vi "vew --scan pipe.vi"() -> ()   [LabVIEW 2010]
uses:
  <vilib>/event_ctls.llb/eventvkey.ctl
  cursor window action.ctl
  cursor winow.ctl
  tale of three indices -- int -- control.ctl
  filter method control.ctl
panel:
  in  "filter method":T1
  in  "step once":bool
  out "Numeric":i32
  out "tale of three indices -- int -- control out":T2={"left"=0, "center"=0, "right"=0, "right most"=0, "left most"=0, "window"=0, "max win factor"=2, "max win"=2, "min win"=2}
  out "norm":dbl
  out "center":cdb
  out "Plot: fragment":cluster{dbl[], dbl[]}[](graph)
  in  "smart filter: span":dbl(slide)=0.1 min=0.0001 max=0.5 step=0.001 scale=0.001..0.5 scale format="%#_2g"
  in  "smart filter: delta":dbl(slide)=0.1 min=0.0005 max=0.1 step=0.0001 scale=0.0001..0.1 scale format="%#_2g"
  in  "scale gauge: Plot: complex plane - filter":dbl(slide)=0.3 min=0.0 max=0.3 step=1e-05 scale=1e-05..0.3 scale format="%#_2g"
  out "Plot: complex plane - filter":cluster{dbl[], dbl[]}[](graph)=[{array[1630 elements], array[1630 elements]}, {[0.4066553079816637, 0.40327728987953354, 0.3931965089365436, 0.37657194509013175, 0.35366577764318885, 0.3248392505398343, 0.2905469753326207, 0.2513297616867779, 0.20780608848872892, 0.16066235006458904, 0.11064203133161113, 0.058533982596904274, 0.005159978916854432, -0.048638239786419776, -0.10201224346646971, -0.15412029220117648, -0.20414061093415437, -0.25128434935829436, -0.29480802255634325, -0.33402523620218605, -0.36831751140939956, -0.39714403851275415, -0.4200502059596971, -0.4366747698061089, -0.44675555074909884, -0.450133568851229, -0.44675555074909884, -0.4366747698061089, -0.420050205959697, -0.3971440385127541, -0.3683175114093995, -0.334025236202186, -0.29480802255634314, -0.25128434935829413, -0.20414061093415412, -0.15412029220117648, -0.10201224346646963, -0.04863823978641969, 0.005159978916854609, 0.05853398259690454, 0.11064203133161105, 0.160662350064589, 0.207806088488729, 0.25132976168677806, 0.2905469753326208, 0.3248392505398345, 0.35366577764318885, 0.3765719450901318, 0.3931965089365437, 0.40327728987953354], [-0.02173913043478265, 0.03195292977291478, 0.08479823411705473, 0.1359633805798755, 0.18464146423708142, 0.23006480263052065, 0.27151704257914155, 0.30834445749658657, 0.33996625704997624, 0.36588374657040623, 0.3856881917657815, 0.399067264704769, 0.40580996941485, 0.40580996941485, 0.39906726470476894, 0.3856881917657815, 0.36588374657040623, 0.33996625704997624, 0.30834445749658657, 0.2715170425791415, 0.23006480263052065, 0.18464146423708136, 0.1359633805798754, 0.08479823411705474, 0.03195292977291471, -0.02173913043478279, -0.07543119064248009, -0.12827649498662014, -0.17944164144944094, -0.22811972510664674, -0.273543063500086, -0.31499530344870685, -0.3518227183661519, -0.38344451791954165, -0.40936200743997164, -0.4291664526353468, -0.4425455255743343, -0.4492882302844153, -0.4492882302844153, -0.44254552557433424, -0.42916645263534686, -0.40936200743997153, -0.38344451791954154, -0.3518227183661518, -0.3149953034487067, -0.27354306350008567, -0.22811972510664671, -0.17944164144944075, -0.12827649498661992, -0.07543119064247988]}, {[-0.08588521013843603, -0.0794706021680707, -0.07305599419770535, -0.06664138622734002, -0.06022677825697468, -0.05381217028660934, -0.04739756231624401, -0.04098295434587867, -0.03456834637551333, -0.02815373840514799, -0.02173913043478265, -0.015324522464417317, -0.008909914494051985, -0.0024953065236866384, 0.003919301446678694, 0.01033390941704404, 0.016748517387409373, 0.023163125357774705, 0.029577733328140052, 0.035992341298505384], [0.4018255934561417, 0.35946912106704926, 0.31711264867795685, 0.2747561762888644, 0.23239970389977196, 0.19004323151067953, 0.14768675912158707, 0.10533028673249467, 0.06297381434340221, 0.020617341954309754, -0.02173913043478265, -0.06409560282387511, -0.10645207521296757, -0.14880854760206003, -0.19116501999115237, -0.23352149238024483, -0.2758779647693373, -0.31823443715842975, -0.3605909095475222, -0.40294738193661456]}, {[0.4018255934561417, 0.35946912106704926, 0.31711264867795685, 0.2747561762888644, 0.23239970389977196, 0.19004323151067953, 0.14768675912158707, 0.10533028673249467, 0.06297381434340221, 0.020617341954309754, -0.02173913043478265, -0.06409560282387511, -0.10645207521296757, -0.14880854760206003, -0.19116501999115237, -0.23352149238024483, -0.2758779647693373, -0.31823443715842975, -0.3605909095475222, -0.40294738193661456], [0.04240694926887073, 0.03599234129850539, 0.029577733328140055, 0.02316312535777472, 0.01674851738740938, 0.01033390941704404, 0.003919301446678708, -0.0024953065236866315, -0.008909914494051971, -0.01532452246441731, -0.02173913043478265, -0.028153738405147982, -0.034568346375513315, -0.04098295434587866, -0.047397562316243994, -0.05381217028660934, -0.06022677825697467, -0.06664138622734, -0.07305599419770535, -0.07947060216807068]}, {[-0.03480491194516355, -0.03153571549706419, -0.02826039650219348, -0.024981001928307045, -0.021699581290264596, -0.018418185369150124, -0.015138864930600241, -0.011863669443142526, -0.008594645797344487, -0.0053338370265733695, -0.002083281030167059, 0.0011549907001868857, 0.004378954350067313, 0.007586595047137542, 0.010775908120375176, 0.01394490035292599, 0.017091591227799845, 0.020214014165629166, 0.023310217753717, 0.02637826696560664], [-0.15235728022815603, -0.15264307469559787, -0.15284705845898403, -0.15296910403510236, -0.15300913514944053, -0.15296712678385516, -0.15284310519220728, -0.1526371478839546, -0.15234938357571062, -0.15197999211080082, -0.15152920434686656, -0.15099730201158656, -0.15038461752660615, -0.14969153379978473, -0.1489184839858907, -0.1480659512158939, -0.1471344682950244, -0.1461246173697867, -0.14503702956413708, -0.14387238458505142]}, {[-0.03913246135316176, -0.03478046636428151, -0.030420320964959106, -0.026054750104140326, -0.021686482121507648, -0.017318247042357023, -0.012952774871420701, -0.008592793886703221, -0.004241028934396603, 9.980027406010505e-05, 0.00442698086171163, 0.008737808481546538, 0.013029589006625965, 0.017299640213825143, 0.021545293460135825, 0.02576389535048096, 0.02995280939600055, 0.03410941766177122, 0.038231122402930216, 0.04231534768818167], [-0.19561963666378376, -0.19600008981485692, -0.19627163553875665, -0.19643410412824466, -0.19648739404574114, -0.19643147198678232, -0.19626637290083468, -0.19599219996945272, -0.19560912454179388, -0.1951173860275308, -0.19451729174722807, -0.19380921674027698, -0.19299360353050807, -0.1920709618496281, -0.1910418683186543, -0.1899069660875451, -0.18866696443325223, -0.1873226383164459, -0.18587482789718943, -0.1843244380098665]}]
  in  "create bin file from dat":bool=TRUE
  in  "# columns in bin file":i32=3
  in  "read freq in":bool=TRUE
  in  "filter window (kHz)":dbl=40.0 caption="(kHz)"
  out "all:max omega":dbl=3099.911666666456
  out "all:min omega":dbl=450.0
  in  "filter  all":bool
  in  "phase is normalized":bool=TRUE
  out "Plot: All":cluster{"all rows":dbl[], "all rows":dbl[]}[](graph)
  in  "cursor bracket: All, data window":T3={"left"=2889.388009121066, "right "=2961.3698154668923, "center"=2923.047912677266, "window"=71.98180634582651, "cursors"=[0, 1, 2], "relative"=1, "absolute"=1, "fixed vertical offset"=2421.6740576496672, "vertical offset"=2421.6740576496672, "skew"=0.0, "default window frac"=0.0, "kind"=enum."symmetric", "skew.left"=0.3, "skew.right"=1.0, "Plot ref"=refnum, "wing order"=enum."back"}
  out "filter w (kHz)":dbl
  out "Char":i16
  in  "file path":path=path "C:/data/RUS/Experiment/ProbeTest/Probe10/Hg1201-4-C199-80K-1/Sweep1/March_2012/032212/201.57400K_900_2100_001_032212.bin"
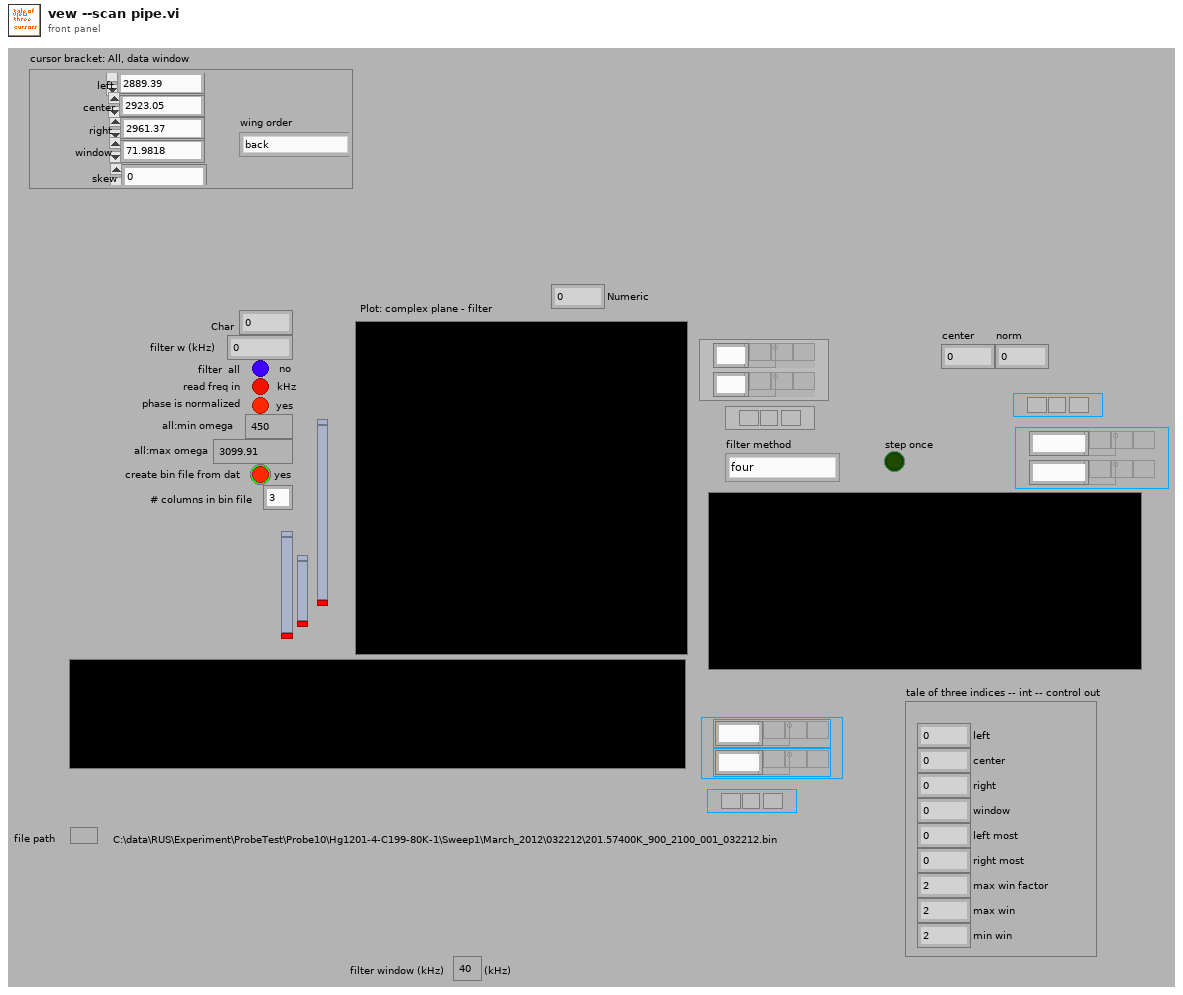
[diagram p1: front panel]
types:
  T1 = typedef "filter method control.ctl" = enum16{"four", "five", "one", "two", "three", "zero", "minus one", "minus two"}
  T2 = typedef "tale of three indices -- int -- control.ctl" = cluster{"left":i32, "center":i32, "right":i32, "right most":i32, "left most":i32, "window":i32, "max win factor":i32, "max win":i32, "min win":i32}
  T3 = typedef "cursor winow.ctl" = cluster{"left":dbl, "right ":dbl, "center":dbl, "window":dbl, "cursors":i32[], "relative":i32, "absolute":i32, "fixed vertical offset":dbl, "vertical offset":dbl, "skew":dbl, "default window frac":dbl, "kind":enum16{"symmetric", "skewed", "fancy"}, "skew.left":dbl, "skew.right":dbl, "Plot ref":refnum<vi>, "wing order":enum16{"forw", "back"}}
  T4 = typedef "eventvkey.ctl" = enum16{"ASCII", "Enter", "Return", "Shift", "Ctrl", "Alt", "Cmd", "Opt", "Caps", "NumLock", "Clear", "Break", "Up", "Down", "Left", "Right", "Insert", "Delete", "Home", "End", "PageUp", "PageDown", "Escape", "Help", "Pause", "ScrollLock", "F1", "F2", "F3", "F4", "F5", "F6", "F7", "F8", "F9", "F10", "F11", "F12", "F13", "F14", "F15", "F16", "F17", "F18", "F19", "F20", "F21", "F22", "F23", "F24", "Play", "VolumeUp", "VolumeDown", "Mute", "Two Byte Char"}
  T5 = typedef "cursor window action.ctl" = enum16{"balance", "h. offset change", "cursor moves", "change center", "change window", "init", "check", "reset", "set y to middle", "idle", "-write all Y", "-write left.X", "-write center.X", "-write right.X", "-write all X", "-change center", "-change window", "-change skew", "-read cursor 2", "-read cursor 1", "-read cursor 0", "-read all cursors", "-reset", "-read plot scale", "-set y to middle", "-Q: center.Y is visible", "-Q: window is visible", "-parse center.Y", "-right left from center", "-left move", "-right move", "-set center.Y", "-empty", "-set cursors to default", "-check", "-write center.Y", "-copy cursor 1", "-copy cursor 0", "-copy cursor 2", "move right", "move left", "shrink", "broaden", "skew up", "skew down", "-write plot scale", "zoom X", "change cen&win"}
  T6 = cluster{"left":dbl, "right ":dbl, "center":dbl, "window":dbl, "cursors":i32[], "relative":i32, "absolute":i32, "fixed vertical offset":dbl, "vertical offset":dbl, "skew":dbl, "default window frac":dbl, "kind":enum16{"symmetric", "skewed", "fancy"}, "skew.left":dbl, "skew.right":dbl, "Plot ref":refnum<vi>, "wing order":enum16{"forw", "back"}}
  T7 = typedef "lveventtype.ctl" = enum32{"Null", "Timeout", "App Instance Close", "App Instance Close?", "Autoscale Range Change", "Cell Edit", "Cell Edit?", "Cursor Grab", "Cursor Grab?", "Cursor Move", "Cursor Release", "Data Change", "Direction Change", "Display State Change", "Drag Ended", "Drag Enter", "Drag Leave", "Drag Over", "Drag Source Update", "Drag Starting", "Drag Starting?", "Drop", "Exec State Change", "Key Down", "Key Down?", "Key Repeat", "Key Repeat?", "Key Up", "Listbox Double Click", "Menu Activation?", "Menu Selection (App)", "Menu Selection? (App)", "Menu Selection (User)", "Mouse Down", "Mouse Down?", "Mouse Enter", "Mouse Leave", "Mouse Move", "Mouse Up", "NI Security User Change (App)", "Pane Size", "Panel Close", "Panel Close?", "Panel Resize", "Plot Attribute Change", "Scale Range Change", "Shortcut Menu Activation?", "Shortcut Menu Selection (App)", "Shortcut Menu Selection? (App)", "Shortcut Menu Selection (User)", "Tree Double Click", "Tree Drag", "Tree Drag?", "Tree Drop", "Tree Drop?", "Tree Item Close", "Tree Item Close?", "Tree Item Open", "Tree Item Open?", "Value Change"}
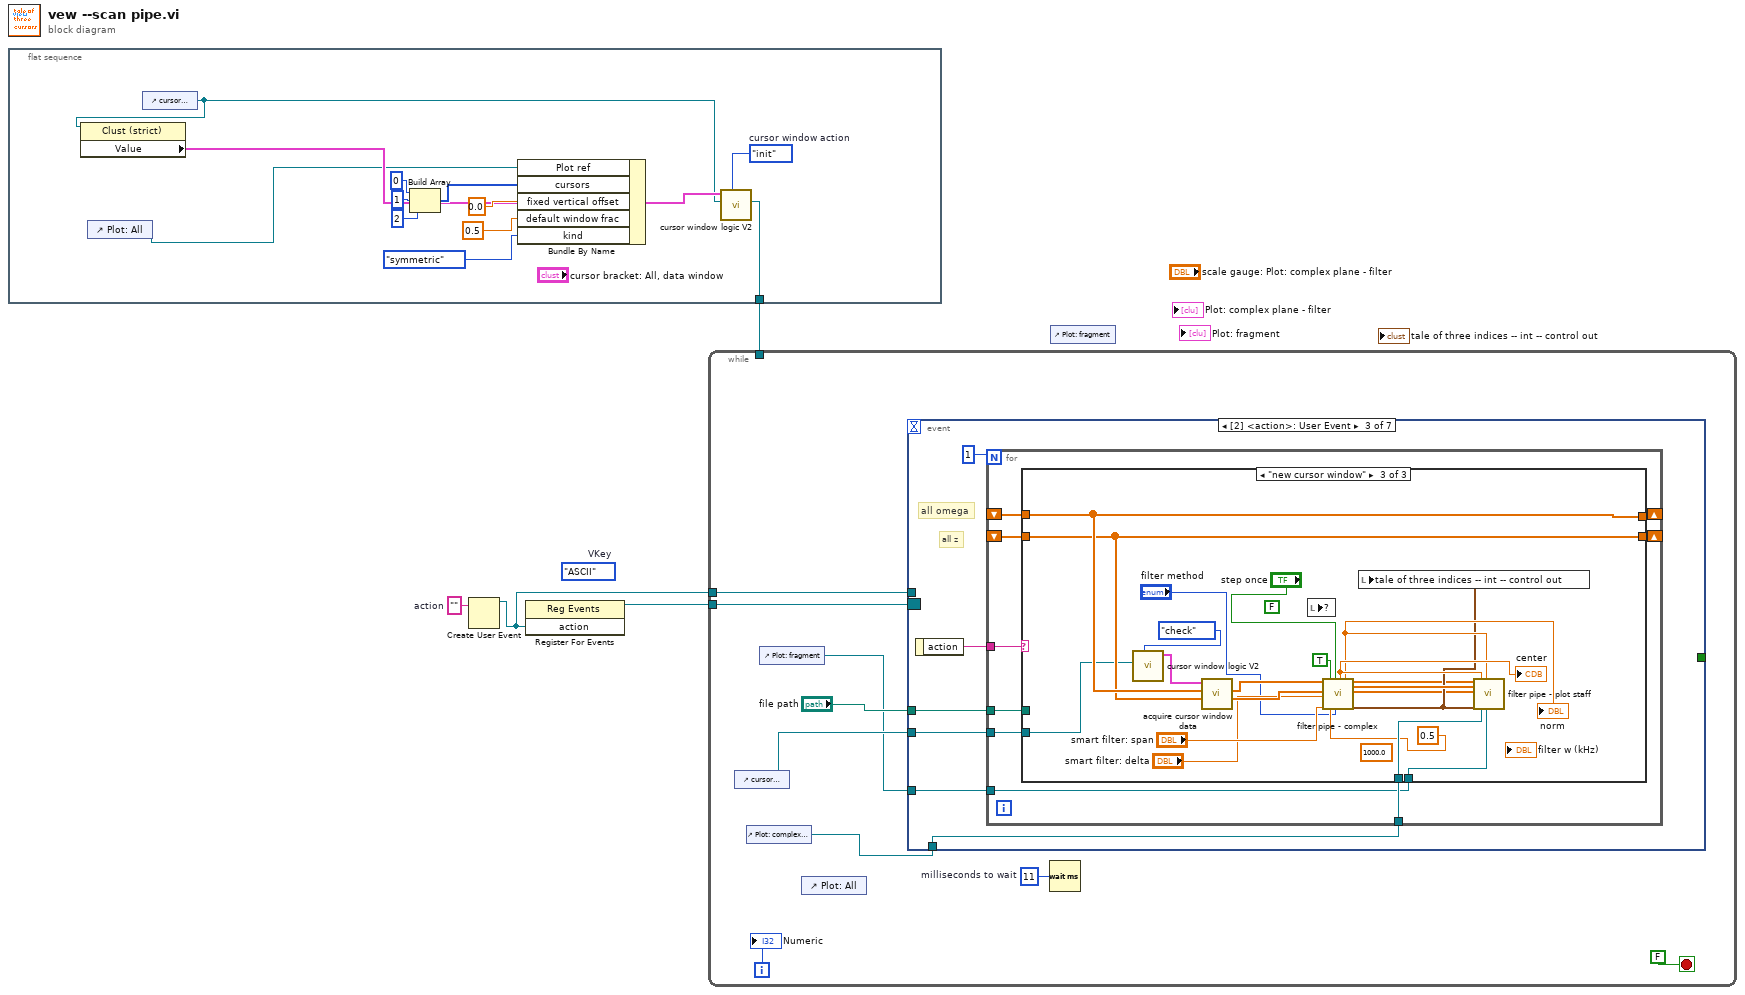
[diagram p0: block diagram]
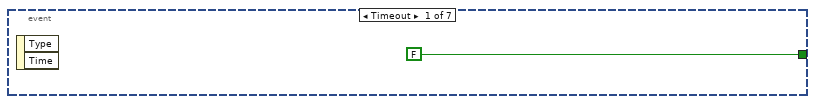
[diagram p2: hidden frame]
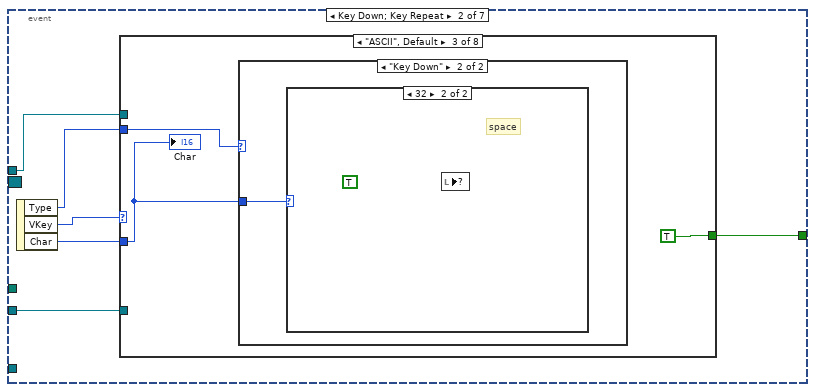
[diagram p3: hidden frame]
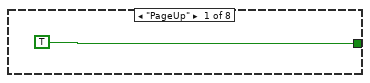
[diagram p4: hidden frame]
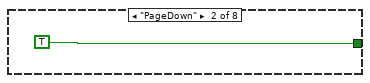
[diagram p5: hidden frame]
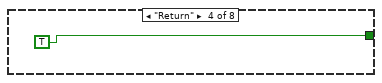
[diagram p8: hidden frame]
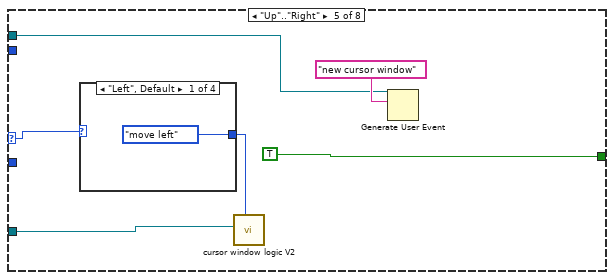
[diagram p9: hidden frame]
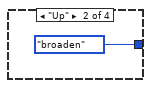
[diagram p10: hidden frame]
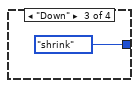
[diagram p11: hidden frame]
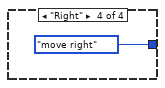
[diagram p12: hidden frame]
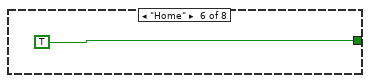
[diagram p13: hidden frame]
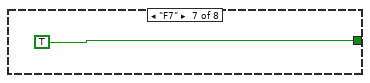
[diagram p14: hidden frame]
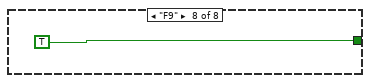
[diagram p15: hidden frame]
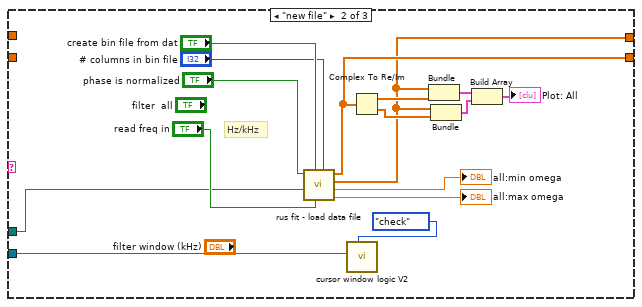
[diagram p17: hidden frame]
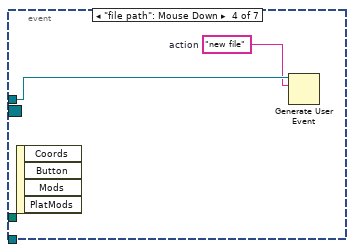
[diagram p18: hidden frame]
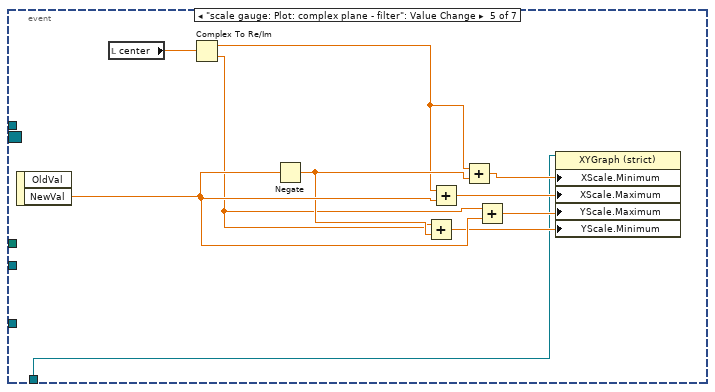
[diagram p19: hidden frame]
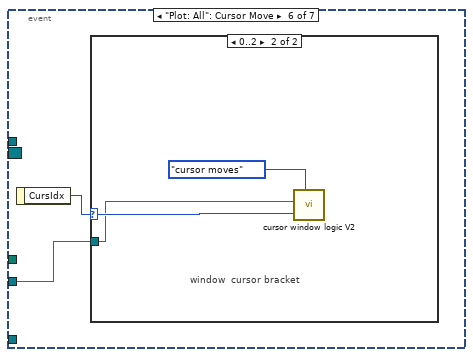
[diagram p20: hidden frame]
diagram:
  (unwired) eventvkey."ASCII"  # VKey
  w3 = ""  # action
  n1 = flat-sequence {
    tunnel: [w5] -> w2
    frame #0 {
      w8 = cursor_window_action."init"  # cursor window action
      n2 = control-ref of="Plot: All"() -> (w7:refnum<vi>)
      n3 = control-ref of="cursor bracket: All, data window"() -> (w6:refnum<vi>)
      n4 = property class="Clust (strict)"(reference=w6) -> ("Value"=w9:T6)  [unwired: 1 in, 2 out]
      n5 = Build Array(0, 1, 2) -> (w16:i32[])
      n6 = Bundle By Name(cluster=w9, "Plot ref"=w7, "cursors"=w16, "fixed vertical offset"=0.0, "default window frac"=0.5 ("fixed vertical offset"), "kind"=enum16{"symmetric", "skewed", "fancy"}."symmetric") -> (w17:T6)
      n7 = call "cursor window logic V2.vi"("cursor window action"=w8, "cursor window in"=w6, "cursor window init"=w17) -> ("cursor window out"=w5:refnum<vi>)  [unwired: 7 in, 1 out]
    }
  }
  n8 = Create User Event(user event datatype=w3) -> (user event=w1:refnum<user-event>)  [unwired: 1 in, 1 out]
  n9 = register-events(w1) -> (reference out=w4:refnum<event-registration>)  [unwired: 2 in, 1 out]
  n10 = while {
    tunnel: w4 -> [w26]
    tunnel: w2 -> [_]
    tunnel: w1 -> [w21]
    i -> [w18]
    stop <- FALSE stop-if-true
    w25 = u32 11  # milliseconds to wait
    n11 = control-ref of="cursor bracket: All, data window"() -> (w22:refnum<vi>)
    n12 = control-ref of="Plot: complex plane - filter"() -> (w20:refnum<vi>)
    n13 = control-ref of="Plot: fragment"() -> (w19:refnum<vi>)
    n14 = control-ref of="Plot: All"() -> ()  [unwired: 1 out]
    n15 = event shown="[2] <action>: User Event" {
      selector: w26 -> [_ _ _ _ _ _ _]
      dyn-events: _ -> [_ _ _ _ _ _ _]
      timeout: _ -> [_ _ _ _ _ _ _]
      tunnel: [FALSE w31 _ _ _ _ _] -> _
      tunnel: "file path" -> [_ _ w58 _ _ _ _]
      tunnel: w22 -> [_ w29 w57 _ _ w120 _]
      tunnel: w21 -> [_ w28 _ w109 _ _ w125]
      tunnel: w20 -> [_ _ w55 _ w110 _ _]
      tunnel: w19 -> [_ _ w54 _ _ _ _]
      event Timeout {
        n16 = event-data() -> ()  [unwired: 1 in, 2 out]
      }
      event Key Down; Key Repeat {
        n17 = event-data() -> ("Type"=w30:T7, "VKey"=w33:T4, "Char"=w32:i16)  [unwired: 1 in]
        n18 = case shown="\"ASCII\", Default" w33 {
          selector: w33 -> [_ _ _ _ w41 _ _ _]
          tunnel: w32 -> [_ _ w37 _ _ _ _ _]
          tunnel: [TRUE TRUE TRUE TRUE TRUE TRUE TRUE TRUE] -> w31
          tunnel: w30 -> [_ _ w36 _ _ _ _ _]
          tunnel: w29 -> [_ _ _ _ w45 _ _ _]
          tunnel: w28 -> [_ _ _ _ w42 _ _ _]
          frame "PageUp" {
          }
          frame "PageDown" {
          }
          frame "ASCII", Default {
            n19 = case shown="\"Key Down\"" w36 {
              tunnel: w37 -> [_ w39]
              frame "Null", Default {
              }
              frame "Key Down" {
                n20 = case shown="32" w39 {
                  frame 0, Default {
                  }
                  frame 32 {
                    (unwired) TRUE
                    # "space"
                    n21 = local read item#-1() -> ()  [unwired: 1 in]
                  }
                }
              }
            }
            "Char" <- w37
          }
          frame "Return" {
          }
          frame "Up".."Right" {
            n22 = case shown="\"Left\", Default" w41 {
              tunnel: [cursor_window_action."move left" ("cursor window action") cursor_window_action."broaden" ("cursor window action") cursor_window_action."shrink" ("cursor window action") cursor_window_action."move right" ("cursor window action")] -> w44
              frame "Left", Default {
              }
              frame "Up" {
              }
              frame "Down" {
              }
              frame "Right" {
              }
            }
            n23 = call "cursor window logic V2.vi"("cursor window action"=w44, "cursor window in"=w45) -> ()  [unwired: 8 in, 2 out]
            n24 = Generate User Event(user event=w42, event data cluster="new cursor window" ("event data")) -> ()  [unwired: 1 in, 2 out]
          }
          frame "Home" {
          }
          frame "F7" {
          }
          frame "F9" {
          }
        }
      }
      event User Event {
        # "all z"
        # "all omega"
        n25 = event-data() -> ("action"=w59:string)  [unwired: 1 in]
        n26 = for {
          N: 1 -> [_]
          tunnel: w59 -> [w68]
          tunnel: w58 -> [w67]
          shift-right: [w66] -> _
          shift-left: _ -> [w63]
          shift-right: [w65] -> _
          shift-left: _ -> [w64]
          tunnel: w57 -> [w62]
          tunnel: w55 -> [w61]
          tunnel: w54 -> [w60]
          n27 = case shown="\"new cursor window\"" w68 {
            tunnel: w67 -> [_ w75 _]
            tunnel: [w69 w74 w104] -> w66
            tunnel: [w70 w73 w105] -> w65
            tunnel: w64 -> [w70 _ w105]
            tunnel: w63 -> [w69 _ w104]
            tunnel: w62 -> [_ w71 w103]
            tunnel: w61 -> [_ _ w99]
            tunnel: w60 -> [_ _ w100]
            frame "False", Default {
            }
            frame "new file" {
              # "Hz/kHz"
              n28 = call "rus fit - load data file.vi"("number of columns in the binary file"="# columns in bin file", "read freq in"="read freq in", "create bin file when only dat file is present"="create bin file from dat", "file path"=w75, "phase is normalized"="phase is normalized") -> ("all:max omega"=→"all:max omega":dbl, "all:min omega"=→"all:min omega":dbl, "omega"=w73:dbl[], "x + iy"=w74:cdb[])  [unwired: 2 in, 1 out]
              n29 = call "cursor window logic V2.vi"("cursor window action"=cursor_window_action."check", "cursor window in"=w71) -> ()  [unwired: 8 in, 2 out]
              n30 = Complex To Re/Im(x + iy=w74) -> (x=w83:dbl[], y=w82:dbl[])
              n31 = Bundle("omega"=w73, w83) -> (w84:cluster{"omega":dbl[], dbl[]})  [unwired: 1 in]
              n32 = Bundle("omega"=w73, w82) -> (w85:cluster{"omega":dbl[], dbl[]})  [unwired: 1 in]
              n33 = Build Array(w84, w85) -> (→"Plot: All":cluster{"omega":dbl[], dbl[]}[])
            }
            frame "new cursor window" {
              (unwired) FALSE
              (unwired) 1000.0 ("fixed vertical offset")
              n34 = call "cursor window logic V2.vi"("cursor window action"=cursor_window_action."check", "cursor window in"=w103) -> ("cursor window out"=w106:T3)  [unwired: 8 in, 1 out]
              n35 = call "acquire cursor window data.vi"("z in"=w104, "omega in"=w105, "cursor window"=w106) -> ("z out"=w102:cdb[], "omega  out"=w101:dbl[])  [unwired: 7 in]
              n36 = local read item#-1() -> ()  [unwired: 1 in]
              n37 = call "filter pipe - complex.vi"("omega  in"=w101, "z in"=w102, "delta"="smart filter: delta", "span"="smart filter: span", "init"=TRUE, "interpolated gamma (kHz)"=0.5 ("fixed vertical offset"), "step once"="step once", "filter method"="filter method") -> ("center"=w97:cdb, "norm"=w96:dbl, "omega out"=w88:dbl[], "z in out"=w91:cdb[], "z out"=w87:cdb[], "tale of three indices -- int -- control out"=w89:T2)  [unwired: 5 in, 1 out]
              "center" <- w97
              "norm" <- w96
              n38 = local write "tale of three indices -- int -- control out"(w89) -> ()
              n39 = call "filter pipe - plot staff.vi"("omega  in"=w88, "zin"=w91, "z out"=w87, "tale of three indices -- int -- control"=w89, "center"=w97, "Plot: complex plane - filter"=w99, "norm"=w96, "Plot: fragment"=w100) -> ()  [unwired: 12 in]
            }
          }
        }
      }
      event "file path": Mouse Down {
        w108 = "new file"  # action
        n40 = event-data() -> ()  [unwired: 1 in, 4 out]
        n41 = Generate User Event(user event=w109, event data cluster=w108) -> ()  [unwired: 1 in, 2 out]
      }
      event "scale gauge: Plot: complex plane - filter": Value Change {
        n42 = event-data() -> ("NewVal"=w118:dbl)  [unwired: 1 in, 1 out]
        n43 = local read "center"() -> (w119:cdb)
        n44 = Complex To Re/Im(x + iy=w119) -> (x=w111:dbl, y=w112:dbl)
        n45 = Negate(x=w118) -> (-x=w117:dbl)
        n46 = Add(x=w112, y=w117) -> (x+y=w113:dbl)
        n47 = Add(x=w111, y=w118) -> (x+y=w115:dbl)
        n48 = Add(x=w111, y=w117) -> (x+y=w116:dbl)
        n49 = Add(x=w112, y=w118) -> (x+y=w114:dbl)
        n50 = property on="Property Node" class="XYGraph (strict)"(reference=w110, "XScale.Minimum"=w116, "XScale.Maximum"=w115, "YScale.Maximum"=w114, "YScale.Minimum"=w113) -> ()  [unwired: 1 in, 2 out]
      }
      event "Plot: All": Cursor Move {
        n51 = event-data() -> ("CursIdx"=w121:i32)  [unwired: 1 in]
        n52 = case shown="0..2" w121 {
          selector: w121 -> [_ w124]
          tunnel: w120 -> [_ w122]
          frame 3..5, Default {
          }
          frame 0..2 {
            # "window  cursor bracket"
            n53 = call "cursor window logic V2.vi"("CursIdx"=w124, "cursor window action"=cursor_window_action."cursor moves", "cursor window in"=w122) -> ()  [unwired: 7 in, 2 out]
          }
        }
      }
      event "Plot: All": Cursor Release {
        n54 = event-data() -> ()  [unwired: 1 in, 1 out]
        n55 = Generate User Event(user event=w125, event data cluster="new cursor window" ("event data")) -> ()  [unwired: 1 in, 2 out]
      }
    }
    n56 = Wait (ms)(milliseconds to wait=w25) -> ()  [unwired: 1 out]
    "Numeric" <- w18
  }
  n57 = control-ref of="Plot: fragment"() -> ()  [unwired: 1 out]
